vi "Super Initialize.vi"() -> ()   [LabVIEW 2013]
uses:
  Cartesian/Functions.ctl
panel:
  in  "Functions 3":T1=[11, 12]
  in  "Functions 2":T1=[11, 12]
  in  "Functions 1":T1=[11, 12]
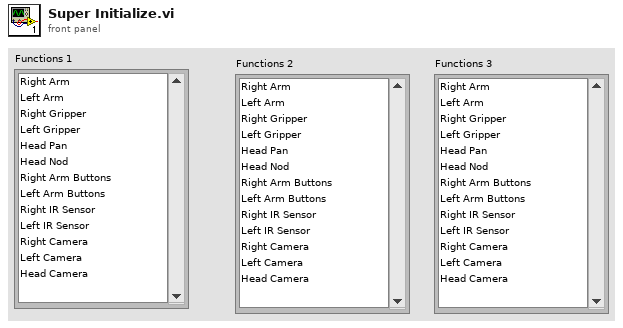
[diagram p1: front panel]
types:
  T1 = typedef "Functions.ctl" = i32[]
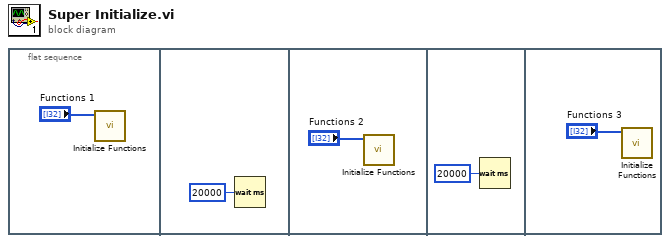
[diagram p0: block diagram]
diagram:
  n1 = flat-sequence {
    frame #0 {
      n2 = call "Initialize Functions.vi"("Functions"="Functions 1") -> ()  [unwired: 10 in, 1 out]
    }
    frame #1 {
      n3 = Wait (ms)(milliseconds to wait=u32 20000) -> ()  [unwired: 1 out]
    }
    frame #2 {
      n4 = call "Initialize Functions.vi"("Functions"="Functions 2") -> ()  [unwired: 10 in, 1 out]
    }
    frame #3 {
      n5 = Wait (ms)(milliseconds to wait=u32 20000) -> ()  [unwired: 1 out]
    }
    frame #4 {
      n6 = call "Initialize Functions.vi"("Functions"="Functions 3") -> ()  [unwired: 10 in, 1 out]
    }
  }
